vi "Read Register.vi"(8 "error in (no error)":errorcluster, 10 "Register Address":u8 format="%.0x", 11 "LINX-ADS1256 in":refnum<class "LINX-ADS1256.lvclass">) -> (0 "error out":errorcluster, 2 "Read Data":u8 format="%.0x", 3 "LINX-ADS1256 out":refnum<class "LINX-ADS1256.lvclass">)   [LabVIEW 2020, in "LINX-ADS1256.lvclass"]
uses:
  LINX-ADS1256.lvclass
  LINX SPI/LINX SPI.lvclass
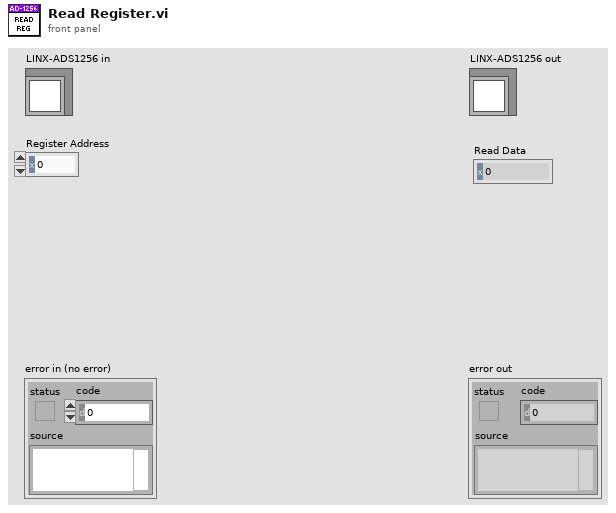
[diagram p1: front panel]
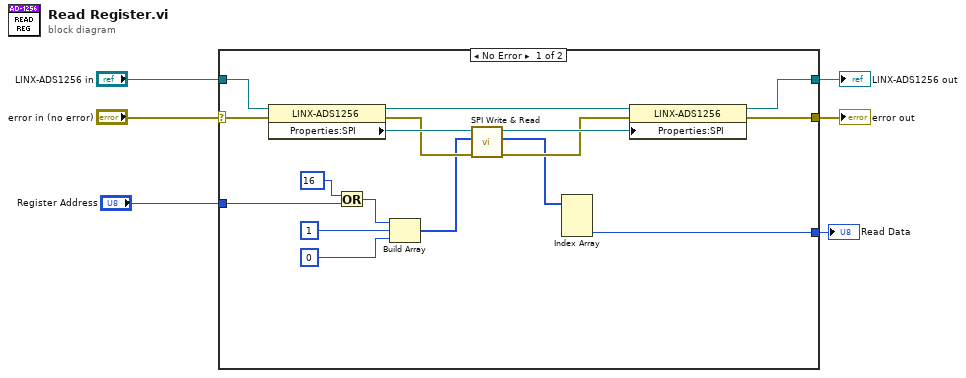
[diagram p0: block diagram]
diagram:
  n1 = case shown="No Error" "error in (no error)" {
    selector: "error in (no error)" -> [w16 w25]
    tunnel: [w15 w25] -> w5
    tunnel: [w17 w24] -> w3
    tunnel: "LINX-ADS1256 in" -> [w23 w24]
    tunnel: [w7 _] -> w2
    tunnel: "Register Address" -> [w14 _]
    frame No Error {
      n2 = property class="LINX-ADS1256"(reference=w23, error in=w16) -> (reference out=w19:refnum<class "LINX-ADS1256.lvclass">, error out=w20:errorcluster, "Properties:SPI"=w22:refnum<class "LINX SPI.lvclass">)
      n3 = Or(x=u8 16 ("SPI Channel"), y=w14) -> (x .or. y?=w12:u8)
      n4 = Build Array(w12, u8 1 ("SPI Channel"), u8 0 ("SPI Channel")) -> (w10:u8[])
      n5 = call "SPI Write & Read.vi"("error in (no error)"=w20, "Data"=w10, "LINX SPI in"=w22) -> ("error out"=w18:errorcluster, "Read Data"=w8:u8[], "LINX SPI out"=w21:refnum<class "LINX SPI.lvclass">)  [unwired: 6 in]
      n6 = Index Array(array=w8) -> (element #3=w7:u8)  [unwired: 3 in, 2 out]
      n7 = property class="LINX-ADS1256"(reference=w19, error in=w18, "Properties:SPI"=w21) -> (reference out=w17:refnum<class "LINX-ADS1256.lvclass">, error out=w15:errorcluster)
    }
    frame Error {
    }
  }
  "error out" <- w5
  "LINX-ADS1256 out" <- w3
  "Read Data" <- w2
